vi "gen_drive_waveform_ramp.vi"(8 "TxRxParams":T1={"sample rate"=1000000.0, "Transmit frequency"=25000.0, "Transmit amplitude"=1.577, "sample rate digital out"=40000.0, "TX cycles"=600, "sample rate DAQ1"=1000000.0, "Receive frequency"=75000.0, "Receive range"=1.0, "TX harmonics"=[50000.0, 75000.0, 100000.0, 125000.0, 150000.0, 175000.0, 200000.0, 225000.0]} {"TX harmonics" format="%#_6p"; "Receive frequency" format="%#_6p"; "sample rate DAQ1" format="%#_6p"; "sample rate digital out" format="%#_6p"; "Transmit frequency" format="%#_6p"; "sample rate" format="%#_6p"}, 9 "ramping cycles":dbl, 10 "ramping?":bool, 11 "no of cycles":dbl=6000.0) -> (0 "signal out":waveform(dbl))   [LabVIEW 2021]
uses:
  <vilib>/Analysis/1siggen.llb/Ramp Pattern by Samples.vi
  <vilib>/measure/NI_MABase.lvlib
  <vilib>/Analysis/NI_AALBase.lvlib
panel:
  out "x/y":dbl
  out "Ramped output waveform":dbl[](graph)
  out "Original output waveform":dbl[](graph)
  out "Ramp Pattern":dbl[](graph)
  out "sample rate (from global)":dbl=500000.0 format="%#_6p"
  out "Transmit amplitude (from global)":dbl=3.3
  out "Transmit frequency (from global)":dbl=25000.0 format="%#_6p"
  out "Sample points per cycle":dbl
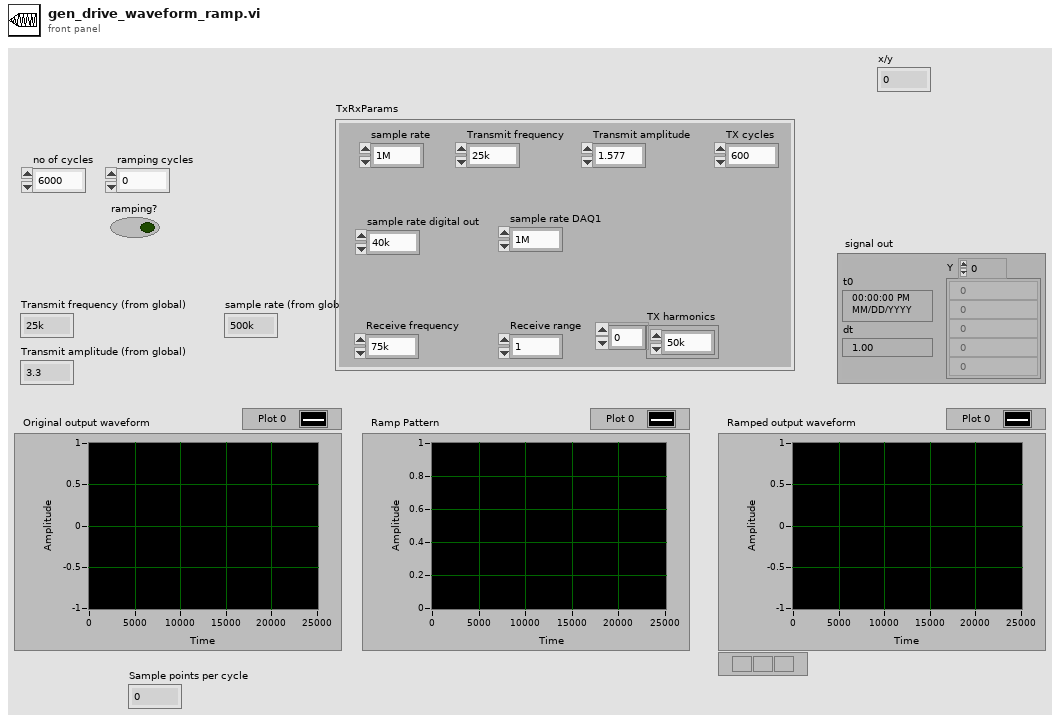
[diagram p1: front panel]
types:
  T1 = cluster{"sample rate":dbl, "Transmit frequency":dbl, "Transmit amplitude":dbl, "sample rate digital out":dbl, "TX cycles":i32, "sample rate DAQ1":dbl, "Receive frequency":dbl, "Receive range":dbl, "TX harmonics":dbl[]}
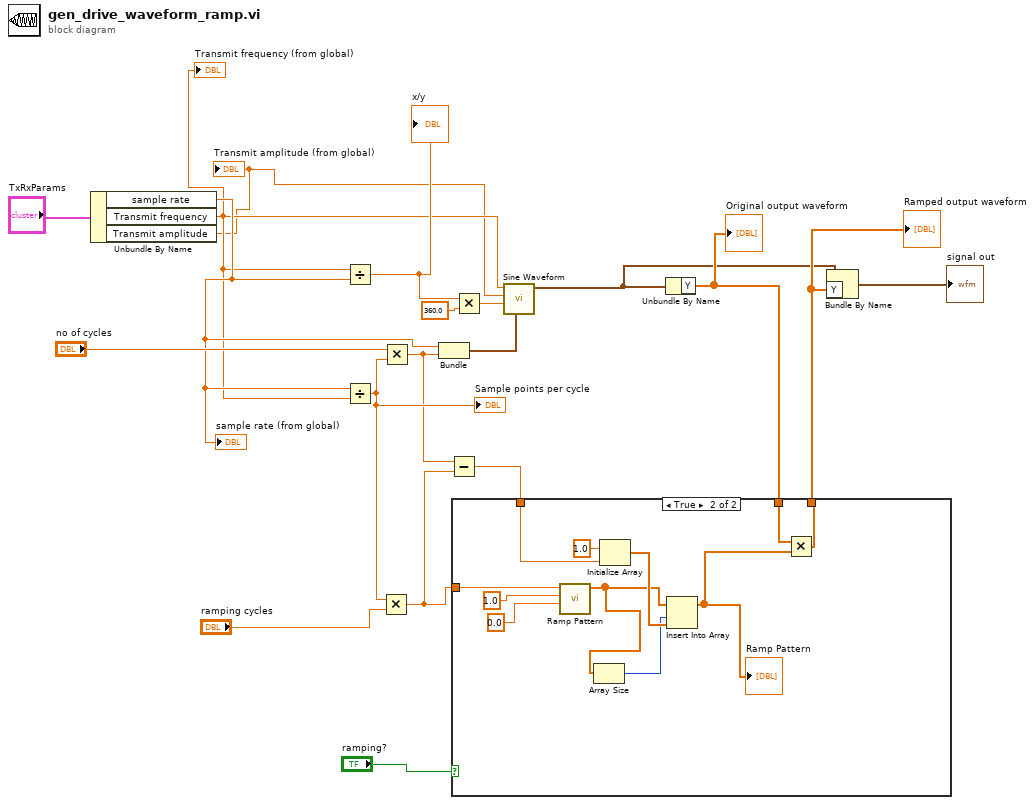
[diagram p0: block diagram]
diagram:
  n1 = Unbundle By Name("TxRxParams") -> ("sample rate"=w3:dbl, "Transmit frequency"=w2:dbl, "Transmit amplitude"=w1:dbl)
  "Transmit frequency (from global)" <- w2
  "Transmit amplitude (from global)" <- w1
  "sample rate (from global)" <- w3
  n2 = Divide(x=w2, y=w3) -> (x/y=w18:dbl)
  "x/y" <- w18
  n3 = Divide(x=w3, y=w2) -> (x/y=w12:dbl)
  "Sample points per cycle" <- w12
  n4 = Multiply(x=w12, y="ramping cycles") -> (x*y=w10:dbl)
  n5 = Multiply(x="no of cycles", y=w12) -> (x*y=w11:dbl)
  n6 = Bundle("sample rate"=w3, w11) -> (w19:cluster{"sample rate":dbl, dbl})  [unwired: 1 in]
  n7 = Subtract(x=w11, y=w10) -> (x-y=w9:dbl)
  n8 = Multiply(x=w18, y=360.0) -> (x*y=w16:dbl)
  n9 = call <vilib>:"Sine Waveform.vi"("sampling info"=w19, "phase"=w16, "amplitude"=w1, "frequency"=w2) -> ("signal out"=w5:waveform(dbl))  [unwired: 6 in, 1 out]
  n10 = Unbundle By Name(w5) -> ("Y"=w7:dbl[])
  "Original output waveform" <- w7
  n11 = case shown="True" "ramping?" {
    tunnel: w10 -> [_ w31]
    tunnel: w7 -> [w20 w30]
    tunnel: [w20 w29] -> w6
    tunnel: w9 -> [_ w26]
    frame False {
    }
    frame True {
      n12 = call-poly <vilib>:"Ramp Pattern.vi"("start"=0.0, "end"=1.0, "samples"=w31) -> ("Ramp Pattern"=w23:dbl[])  [unwired: 7 in, 1 out]
      n13 = Array Size(array=w23) -> (size(s)=w22:i32)
      n14 = Initialize Array(1.0 ("element"), w26) -> (w24:dbl[])
      n15 = Insert Into Array(array=w23, index=w22, new element=w24) -> (w21:dbl[])
      "Ramp Pattern" <- w21
      n16 = Multiply(x=w30, y=w21) -> (x*y=w29:dbl[])
    }
  }
  "Ramped output waveform" <- w6
  n17 = Bundle By Name(cluster=w5, "Y"=w6) -> (→"signal out":waveform(dbl))
